vi "Delete_Table_v2.vi"(6 "Auto?":bool, 8 "error in (no error)":errorcluster, 11 "Ref In":T1={"MS SQL Connection"=refnum, "UDL File"=path "", "Time"="", "DCODE"="", "WIP+1"=0, "MC No?"=0, "POKAYOKE?"=FALSE, "Expected Result"="", "Result [Status]"="", "Clock"=0.0, "RFID"="", "WIP Queue"=refnum, "TS Parameter"={"ProfitCenterCode"="", "LineCode"="", "WorkOrderNumber"="", "Model"="", "Model_with_Prefix"="", "VendorCode"="", "SetParameterDateCode"="", "PokaYoke"=0, "Target"=1, "Live_DateCode"="", "CustomerPartNumber"="", "Hand"="", "sBarcode"=FALSE, "FCA"=0, "Ent_Stamp"=timestamp(0 s since 1904-01-01), "STS_CD"=0.0}, "Data_Queue"=[], "RFID Serial No."=""} {"TS Parameter"."FCA" format="%01d"; "TS Parameter"."Target" min=1 max=100000; "TS Parameter"."PokaYoke" min=0 max=1}) -> (0 "error out":errorcluster)   [LabVIEW 2020]
uses:
  Controls/TD SQL.ctl
  <vilib>/addons/database/Connection.llb/Conn ObjectReference.ctl
  Controls/WIP_State.ctl
  Controls/TS_Parameter.ctl
  MS SQL/MS_Global.vi
  <vilib>/addons/database/NI_Database_API.lvlib
  <vilib>/addons/database/Recordset.llb/Rec Save Format.ctl
  <vilib>/addons/database/Recordset.llb/Rec Destroy - Connection.vi
  <vilib>/addons/database/Recordset.llb/Rec Save Recordset To File (R).vi
  <vilib>/addons/database/Connection.llb/Conn Execute.vi
panel:
  out "Array":string[](array[string])
  out "Data Delete In Process...":dbl(slide) scale=0.0..3000.0
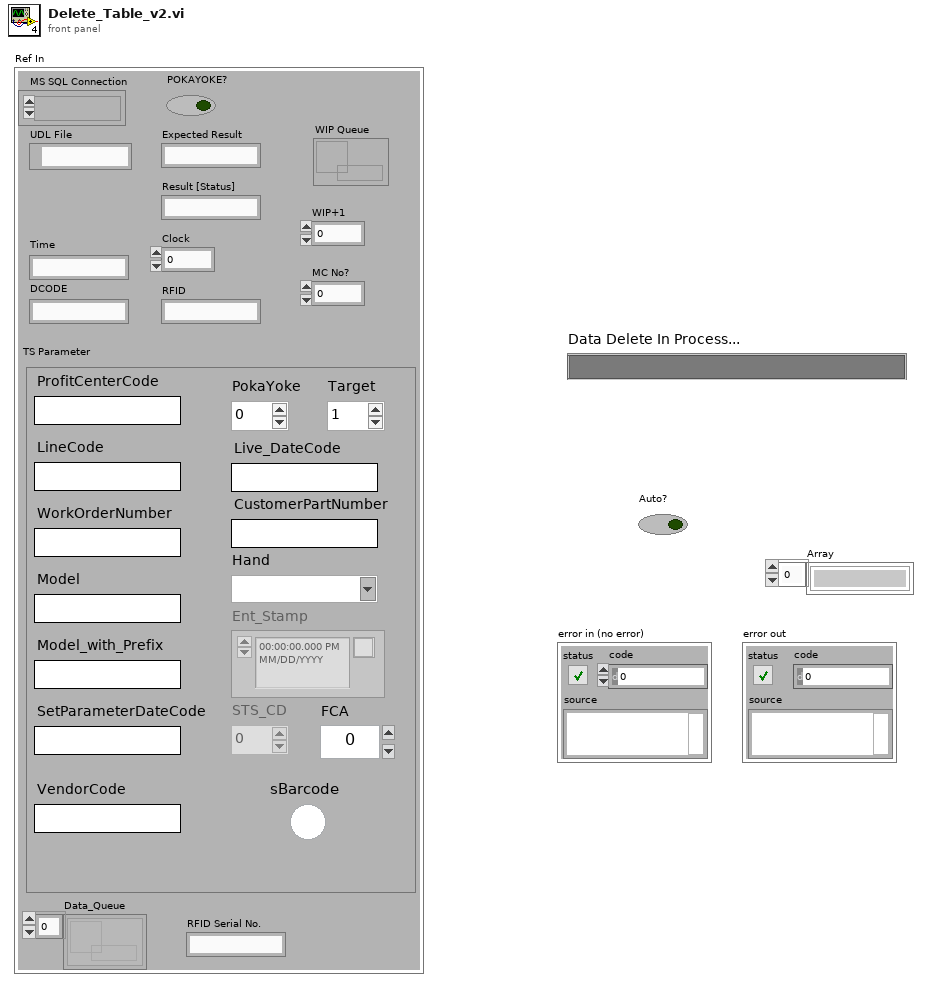
[diagram p1: front panel]
types:
  T1 = typedef "TD SQL.ctl" = cluster{"MS SQL Connection":T2, "UDL File":path, "Time":string, "DCODE":string, "WIP+1":i64, "MC No?":i32, "POKAYOKE?":bool, "Expected Result":string, "Result [Status]":string, "Clock":dbl, "RFID":string, "WIP Queue":refnum<queue>, "TS Parameter":T3, "Data_Queue":refnum<queue>[], "RFID Serial No.":string}
  T2 = typedef "NI_Database_API.lvlib/Conn ObjectReference.ctl" = refnum<k1>
  T3 = typedef "TS_Parameter.ctl" = cluster{"ProfitCenterCode":string, "LineCode":string, "WorkOrderNumber":string, "Model":string, "Model_with_Prefix":string, "VendorCode":string, "SetParameterDateCode":string, "PokaYoke":i32, "Target":i32, "Live_DateCode":string, "CustomerPartNumber":string, "Hand":string, "sBarcode":bool, "FCA":i32, "Ent_Stamp":timestamp, "STS_CD":dbl}
  T4 = typedef "NI_Database_API.lvlib/Rec Save Format.ctl" = enum16{"ADTG", "XML"}
  T5 = typedef "NI_Database_API.lvlib/Rec ObjectReference.ctl" = refnum<k1>
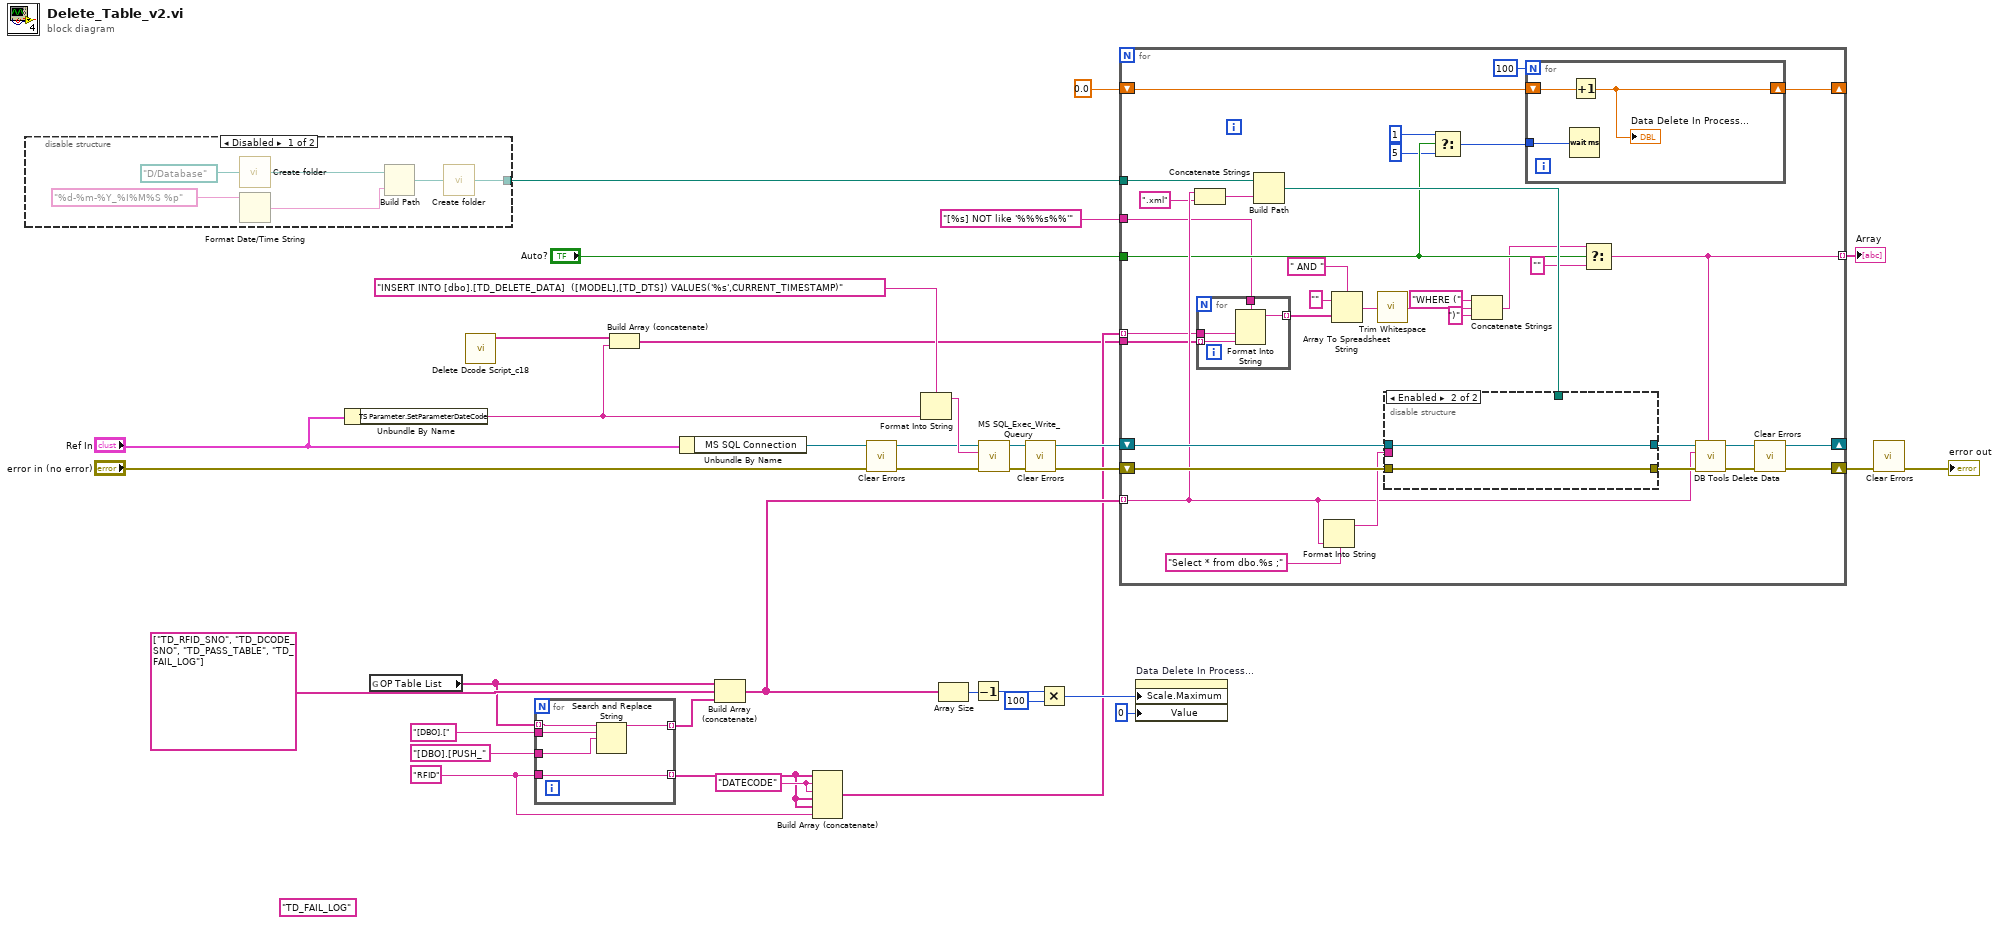
[diagram p0: block diagram]
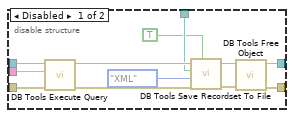
[diagram p3: hidden frame]
diagram:
  (unwired) "TD_FAIL_LOG" ("String")
  w13 = "DATECODE" ("String")
  w3 = "RFID" ("String")
  n1 = disable-structure shown="Disabled" {
    disable-tunnel: [w35 _] -> w32
    frame Disabled {
      n2 = call <userlib>:"Create folder.vi"("Path In"=path "D:/Database") -> ("Path out"=w39:path)  [unwired: 14 in]
      n3 = Format Date/Time String(time format string (%c)="%d-%m-%Y_%I%M%S %p") -> (date/time string=w37:string)  [unwired: 2 in]
      n4 = Build Path(base path=w39, name or relative path=w37) -> (appended path=w36:path)
      n5 = call <userlib>:"Create folder.vi"("Path In"=w36) -> ("Path out"=w35:path)  [unwired: 14 in]
    }
    frame Enabled {
    }
  }
  n6 = Unbundle By Name("Ref In") -> ("TS Parameter.SetParameterDateCode"=w1:string)
  n7 = global read "MS_Global.vi" "OP Table List"() -> (w14:string[])
  n8 = call "Delete Dcode Script_c18.vi"() -> ("Date Codes"=w10:string[])  [unwired: 11 in]
  n9 = for {
    tunnel: w14 -> [w44] mode=indexing
    tunnel: [w45] -> w11 mode=indexing
    tunnel: w3 -> [w45]
    tunnel: "[DBO].[" ("string") -> [w43]
    tunnel: [w41] -> w4 mode=indexing
    tunnel: "[DBO].[PUSH_" ("string") -> [w42]
    n10 = Search and Replace String(input string=w44, search string=w43, replace string=w42) -> (result string=w41:string)  [unwired: 5 in, 3 out]
  }
  n11 = Build Array (concatenate)(w10, w1) -> (w8:string[])
  n12 = Unbundle By Name("Ref In") -> ("MS SQL Connection"=w21:T2)
  n13 = Build Array (concatenate)(w14, string[] ["TD_RFID_SNO", "TD_DCODE_SNO", "TD_PASS_TABLE", "TD_FAIL_LOG"] ("tables"), w4) -> (w15:string[])
  n14 = Build Array (concatenate)(w11, w13, w13, w11, w11, w3) -> (w12:string[])
  n15 = call <vilib>:"Clear Errors.vi"("error in (no error)"="error in (no error)") -> ("error out"=w19:errorcluster)  [unwired: 5 in, 1 out]
  n16 = Format Into String(format string="INSERT INTO [dbo].[TD_DELETE_DATA]  ([MODEL],[TD_DTS]) VALUES('%s',CURRENT_TIMESTAMP)" ("String"), w1) -> (resulting string=w22:string)  [unwired: 2 in, 1 out]
  n17 = Array Size(array=w15) -> (size(s)=w26:i32)
  n18 = Decrement(x=w26) -> (x-1=w30:i32)
  n19 = call "MS SQL_Exec_Write_Queury.vi"("error in (no error)"=w19, "Query"=w22, "Refnum in"=w21) -> ("error out"=w18:errorcluster, "Refnum out"=w20:T2)  [unwired: 7 in]
  n20 = call <vilib>:"Clear Errors.vi"("error in (no error)"=w18) -> ("error out"=w17:errorcluster)  [unwired: 5 in, 1 out]
  n21 = Multiply(x=w30, y=100) -> (x*y=w29:i32)
  n22 = for {
    tunnel: w15 -> [w71] mode=indexing
    shift-right: [w64] -> w34
    shift-left: w17 -> [w76]
    shift-right: [w79] -> _
    shift-left: w20 -> [w78]
    tunnel: w32 -> [w72]
    shift-right: [w66] -> _
    shift-left: 0.0 ("Delete In Process...") -> [w65]
    tunnel: w12 -> [w50] mode=indexing
    tunnel: "Auto?" -> [w62]
    tunnel: "[%s] NOT like '%%%s%%'" ("SQL query") -> [w51]
    tunnel: w8 -> [w49]
    tunnel: [w47] -> w7 mode=indexing
    n23 = Concatenate Strings(w71, ".xml" ("string")) -> (w69:string)
    n24 = for {
      tunnel: w51 -> [w83]
      tunnel: w50 -> [w82]
      tunnel: w49 -> [w81] mode=indexing
      tunnel: [w80] -> w56 mode=indexing
      n25 = Format Into String(format string=w83, w82, w81) -> (resulting string=w80:string)  [unwired: 2 in, 1 out]
    }
    n26 = Build Path(base path=w72, name or relative path=w69) -> (appended path=w68:path)
    n27 = Format Into String(format string="Select * from dbo.%s ;" ("SQL query"), w71) -> (resulting string=w73:string)  [unwired: 2 in, 1 out]
    n28 = Array To Spreadsheet String(delimiter (Tab)=" AND ", array=w56, 3:"" ("format string")) -> (spreadsheet string=w52:string)
    n29 = call <vilib>:"Trim Whitespace.vi"("string"=w52) -> ("trimmed string"=w53:string)  [unwired: 1 in]
    n30 = disable-structure shown="Enabled" {
      disable-tunnel: w78 -> [w93 w97]
      disable-tunnel: [w90 w97] -> w77
      disable-tunnel: w76 -> [w89 w96]
      disable-tunnel: [w88 w96] -> w75
      disable-tunnel: w73 -> [w87 _]
      disable-tunnel: w68 -> [w86 _]
      frame Disabled {
        n31 = call-poly <vilib>:"DB Tools Execute Query.vi"("error in (no error)"=w89, "SQL query"=w87, "connection reference"=w93) -> ("error out"=w94:errorcluster, "recordset reference"=w95:T5)  [unwired: 5 in]
        n32 = call-poly <vilib>:"DB Tools Save Recordset To File.vi"("overwrite? (F)"=TRUE, "error in (no error)"=w94, "save format (XML)"=Rec_Save_Format."XML", "file name"=w86, "recordset reference"=w95) -> ("error out"=w92:errorcluster, "recordset reference out"=w91:T5)  [unwired: 3 in]
        n33 = call-poly <vilib>:"DB Tools Free Object.vi"("error in (no error)"=w92, "recordset reference"=w91) -> ("error out"=w88:errorcluster, "connection reference"=w90:T2)  [unwired: 8 in]
      }
      frame Enabled {
      }
    }
    n34 = Select(t=u32 1 ("milliseconds to wait"), s=w62, f=u32 5 ("milliseconds to wait")) -> (s? t:f=w59:u32)
    n35 = Concatenate Strings("WHERE (" ("string"), w53, ")" ("string")) -> (w48:string)
    n36 = for {
      N: 100 -> [_]
      shift-right: [w99] -> w66
      shift-left: w65 -> [w100]
      tunnel: w59 -> [w98]
      n37 = Wait (ms)(milliseconds to wait=w98) -> ()  [unwired: 1 out]
      n38 = Increment(x=w100) -> (x+1=w99:dbl)
      "Data Delete In Process..." <- w99
    }
    n39 = Select(t=w48, s=w62, f="") -> (s? t:f=w47:string)
    n40 = call <vilib>:"DB Tools Delete Data.vi"("condition"=w47, "error in (no error)"=w75, "table"=w71, "connection reference"=w77) -> ("error out"=w46:errorcluster, "connection reference out"=w79:T2)  [unwired: 6 in]
    n41 = call <vilib>:"Clear Errors.vi"("error in (no error)"=w46) -> ("error out"=w64:errorcluster)  [unwired: 5 in, 1 out]
  }
  "Array" <- w7
  n42 = property on="Data Delete In Process..." class="Slide (strict)"("Scale.Maximum"=w29, "Value"=u8 0 ("Delete In Process...")) -> ()  [unwired: 2 in, 2 out]
  n43 = call <vilib>:"Clear Errors.vi"("error in (no error)"=w34) -> ("error out"=→"error out":errorcluster)  [unwired: 5 in, 1 out]
